vi "Apply.vi"(8 "error in (no error)":errorcluster, 11 "FGen PXI Base CFG in":refnum<class "FGen PXI Base CFG.lvclass">) -> (0 "error out":errorcluster, 3 "FGen PXI Base CFG out":refnum<class "FGen PXI Base CFG.lvclass">)   [LabVIEW 2023, in "FGen PXI Base CFG.lvlib" / "FGen PXI Base CFG.lvclass"]
uses:
  FGen PXI Base CFG.lvclass
  FGen PXI Base CFG.lvclass/FGen PXI Base CFG.ctl
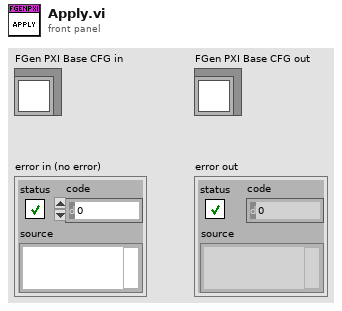
[diagram p1: front panel]
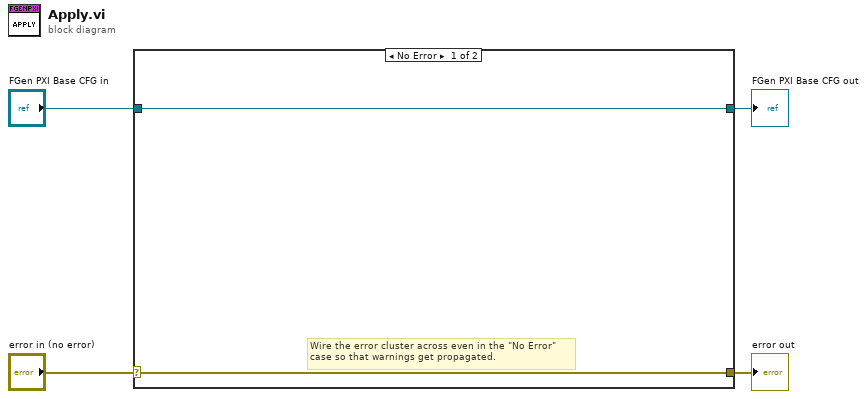
[diagram p0: block diagram]
diagram:
  n1 = case shown="No Error" "error in (no error)" {
    selector: "error in (no error)" -> [w5 w8]
    tunnel: [w5 w8] -> w3
    tunnel: [w6 w7] -> w1
    tunnel: "FGen PXI Base CFG in" -> [w6 w7]
    frame No Error {
      # "Wire the error cluster across even in the \"No Error\"\ncase so that warnings get propagated."
    }
    frame Error {
    }
  }
  "error out" <- w3
  "FGen PXI Base CFG out" <- w1
